vi "ReadVoltageDaq.vi"() -> ()   [LabVIEW 2017]
panel:
  in  "milliseconds to wait":u32
  out "Waveform Graph":cluster{i32, "milliseconds to wait":u32, dbl[]}(graph)
  in  "stop":bool
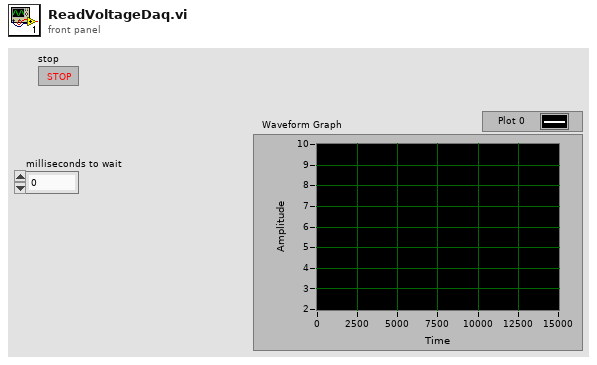
[diagram p1: front panel]
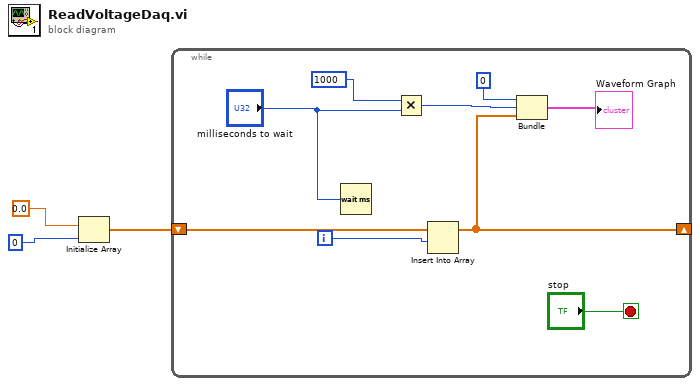
[diagram p0: block diagram]
diagram:
  n1 = Initialize Array(0.0 ("element"), 0 ("dimension size")) -> (w1:dbl[])
  n2 = while {
    shift-right: [w5] -> _
    shift-left: w1 -> [w11]
    i -> [w10]
    stop <- "stop" stop-if-true
    n3 = Wait (ms)(milliseconds to wait="milliseconds to wait") -> ()  [unwired: 1 out]
    n4 = Multiply(x=1000, y="milliseconds to wait") -> (x*y=w4:u32)
    n5 = Insert Into Array(array=w11, index=w10) -> (w5:dbl[])  [unwired: 1 in]
    n6 = Bundle(0, w4, w5) -> (→"Waveform Graph":cluster{i32, u32, dbl[]})  [unwired: 1 in]
  }
